vi "Report Strings.vi"(8 "error in":errorcluster, 10 "data in":T1(array[cluster]), 11 "vi ref in":refnum<vi>) -> (0 "error out":errorcluster, 2 "test jsons out":string[](array[string]), 3 "ats jsons out":string[](array[string]))   [LabVIEW 2019]
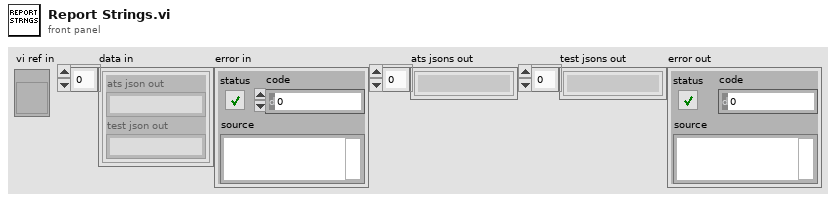
[diagram p1: front panel]
types:
  T1 = cluster{"ats json out":string, "test json out":string}[]
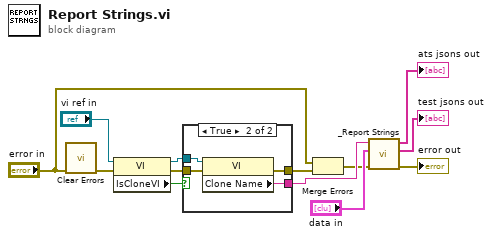
[diagram p0: block diagram]
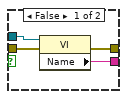
[diagram p2: hidden frame]
diagram:
  n1 = call <vilib>:"Clear Errors.vi"("error in (no error)"="error in") -> ("error out"=w8:errorcluster)  [unwired: 5 in, 1 out]
  n2 = property class="VI"(reference="vi ref in", error in=w8) -> (reference out=w12:refnum<vi>, error out=w13:errorcluster, "IsCloneVI"=w10:bool)
  n3 = case shown="True" w10 {
    tunnel: w12 -> [w17 w21]
    tunnel: [w16 w20] -> w9
    tunnel: [w14 w19] -> w7
    tunnel: w13 -> [w15 w18]
    frame False {
      n4 = property class="VI"(reference=w17, error in=w15) -> (error out=w16:errorcluster, "Name"=w14:string)  [unwired: 1 out]
    }
    frame True {
      n5 = property class="VI"(reference=w21, error in=w18) -> (error out=w20:errorcluster, "Clone Name"=w19:string)  [unwired: 1 out]
    }
  }
  n6 = Merge Errors("error in", w9) -> (w4:errorcluster)
  n7 = call "_Report Strings.vi"("error in"=w4, "data in"="data in", "vi name in"=w7) -> ("error out"=→"error out":errorcluster, "test jsons out"=→"test jsons out":string[], "ats jsons out"=→"ats jsons out":string[])  [unwired: 6 in]
